vi "BFS.vi"(2 "Start (0, 0)":T1, 3 "Visited":bool[][](array[boolean]), 4 "Data":bool[][](array[boolean])) -> (0 "Valid Coordinates":T1[](array[typedef]), 1 "Visited Out":bool[][](array[boolean]))   [LabVIEW 2018, in "Video Cam Processor.lvclass"]
uses:
  Video Cam Processor.lvclass
  Private/Hull Point STYP.ctl
panel:
  out "Queue Status":i32(slide) scale=0.0..307200.0
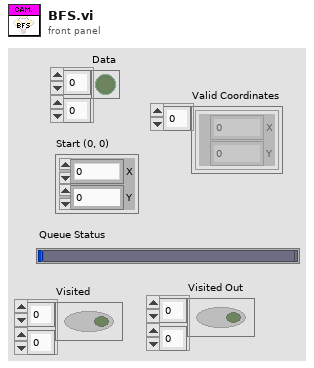
[diagram p1: front panel]
types:
  T1 = typedef "Video Cam Processor.lvclass/Hull Point STYP.ctl" = cluster{"X":i32, "Y":i32}
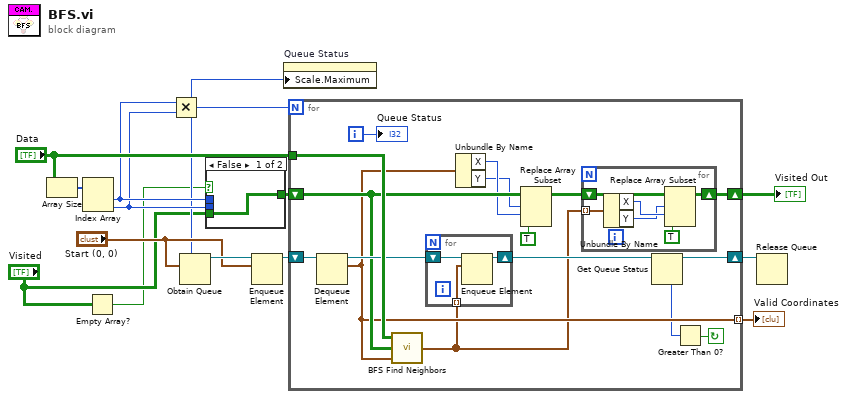
[diagram p0: block diagram]
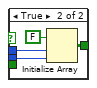
[diagram p2: hidden frame]
diagram:
  n1 = Array Size(array="Data") -> (size(s)=w9:i32[])
  n2 = Index Array(array=w9) -> (element #1=w7:i32, element #2=w6:i32)  [unwired: 2 in]
  n3 = Empty Array?(array="Visited") -> (empty?=w1:bool)
  n4 = Multiply(x=w7, y=w6) -> (x*y=w4:i32)
  n5 = Obtain Queue(max queue size (-1, unlimited)=w4, element data type="Start (0, 0)") -> (queue out=w14:refnum<queue>)  [unwired: 3 in, 2 out]
  n6 = case shown="False" w1 {
    tunnel: [w15 w18] -> w10
    tunnel: w7 -> [_ w17]
    tunnel: w6 -> [_ w16]
    tunnel: "Visited" -> [w15 _]
    frame False {
    }
    frame True {
      n7 = Initialize Array(FALSE, w17, w16) -> (w18:bool[][])
    }
  }
  n8 = Enqueue Element(queue=w14, element="Start (0, 0)") -> (queue out=w13:refnum<queue>)  [unwired: 2 in, 2 out]
  n9 = property on="Queue Status" class="Slide (strict)"("Scale.Maximum"=w4) -> ()  [unwired: 2 in, 2 out]
  n10 = for {
    N: w4 -> [_]
    shift-right: [w26] -> w5
    shift-left: w13 -> [w35]
    tunnel: "Data" -> [w34]
    shift-right: [w20] -> w3
    shift-left: w10 -> [w32]
    tunnel: [w28] -> w8 mode=indexing
    i -> [w23]
    stop <- w24 continue-if-true
    n11 = Dequeue Element(queue=w35) -> (queue out=w33:refnum<queue>, element=w28:T1)  [unwired: 2 in, 2 out]
    n12 = call "BFS Find Neighbors.vi"("Coordinate (0, 0)"=w28, "Visited"=w32, "Data"=w34) -> ("Connected Neighbors"=w21:T1[])
    n13 = for {
      tunnel: w21 -> [w44] mode=indexing
      shift-right: [w42] -> w27
      shift-left: w33 -> [w43]
      n14 = Enqueue Element(queue=w43, element=w44) -> (queue out=w42:refnum<queue>)  [unwired: 2 in, 2 out]
    }
    n15 = Unbundle By Name(w28) -> ("X"=w31:i32, "Y"=w30:i32)
    n16 = Replace Array Subset(array=w32, new element=TRUE ("new element/subarray"), index (row)=w30, index (col)=w31) -> (w22:bool[][])
    n17 = for {
      shift-right: [w40] -> w20
      shift-left: w22 -> [w41]
      tunnel: w21 -> [w39] mode=indexing
      n18 = Unbundle By Name(w39) -> ("X"=w38:i32, "Y"=w37:i32)
      n19 = Replace Array Subset(array=w41, new element=TRUE ("new element/subarray"), index (row)=w37, index (col)=w38) -> (w40:bool[][])
    }
    n20 = Get Queue Status(queue=w27) -> (queue out=w26:refnum<queue>, # elements in queue=w25:i32)  [unwired: 2 in, 6 out]
    n21 = Greater Than 0?(x=w25) -> (x > 0?=w24:bool)
    "Queue Status" <- w23
  }
  "Valid Coordinates" <- w8
  "Visited Out" <- w3
  n22 = Release Queue(queue=w5) -> ()  [unwired: 2 in, 3 out]
